vi "PayneHW1.vi"() -> ()   [LabVIEW 2011]
panel:
  out "Units":string
  in  "stop":bool
  in  "Unit Selector":u16(ring) items=["Celsius", "Kelvin", "Fahrenheit"]
  in  "Voltage":dbl(slide) scale=0.0..4.0
  out "Temperature":dbl(slide) scale=-350.0..600.0
  out "Invalid Range Danger":bool
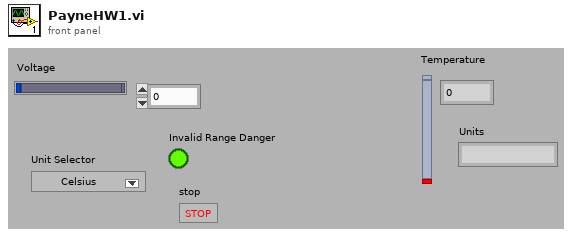
[diagram p1: front panel]
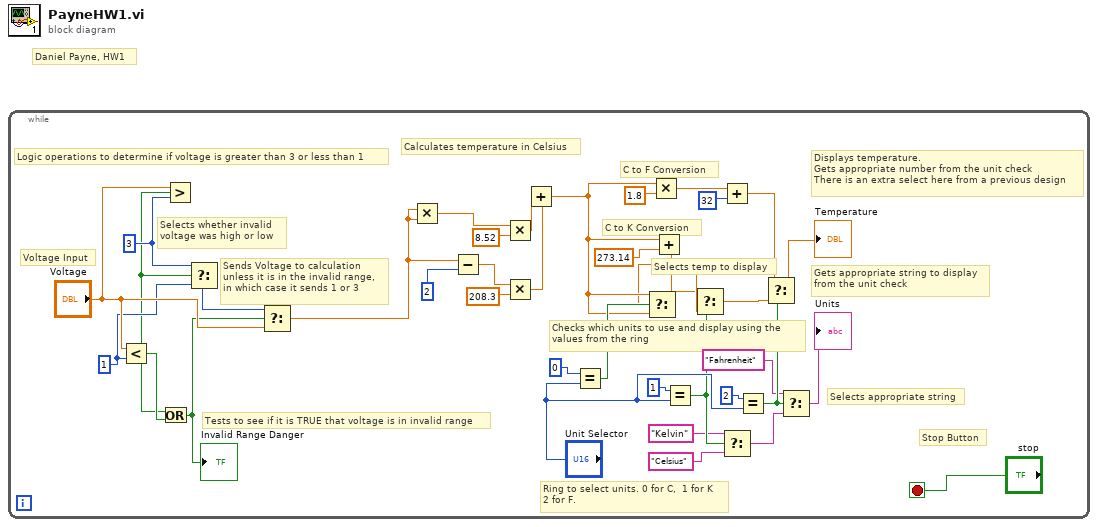
[diagram p0: block diagram]
diagram:
  # "Daniel Payne, HW1"
  n1 = while {
    stop <- "stop" stop-if-true
    w26 = 3
    w25 = 1
    # "Selects temp to display"
    # "C to F Conversion"
    # "C to K Conversion"
    # "Stop Button"
    # "Selects appropriate string"
    # "Displays temperature. \nGets appropriate number from the unit check \nThere is an extra select here from a previous design"
    # "Gets appropriate string to display\nfrom the unit check"
    # "Checks which units to use and display using the\nvalues from the ring"
    # "Ring to select units. 0 for C,  1 for K\n2 for F."
    # "Calculates temperature in Celsius"
    # "Selects whether invalid \nvoltage was high or low"
    # "Sends Voltage to calculation\nunless it is in the invalid range, \nin which case it sends 1 or 3"
    # "Tests to see if it is TRUE that voltage is in invalid range"
    # "Logic operations to determine if voltage is greater than 3 or less than 1"
    # "Voltage Input"
    n2 = Less?(x="Voltage", y=w25) -> (x < y?=w38:bool)
    n3 = Greater?(x="Voltage", y=w26) -> (0:w24:bool)
    n4 = Or(x=w24, y=w38) -> (x .or. y?=w29:bool)
    "Invalid Range Danger" <- w29
    n5 = Select(t=w26, s=w24, f=w25) -> (s? t:f=w27:i32)
    n6 = Select(t=w27, s=w29, f="Voltage") -> (s? t:f=w28:dbl)
    n7 = Multiply(x=w28, y=w28) -> (x*y=w34:dbl)
    n8 = Subtract(x=w28, y=2) -> (x-y=w36:dbl)
    n9 = Multiply(x=w34, y=8.52) -> (x*y=w31:dbl)
    n10 = Multiply(x=w36, y=208.3) -> (x*y=w32:dbl)
    n11 = Add(x=w31, y=w32) -> (x+y=w14:dbl)
    n12 = Equal?(x=0, y="Unit Selector") -> (x = y?=w20:bool)
    n13 = Select(t=w14, s=w20, f=w14) -> (s? t:f=w13:dbl)
    n14 = Multiply(x=w14, y=1.8) -> (x*y=w16:dbl)
    n15 = Add(x=w14, y=273.14) -> (x+y=w12:dbl)
    n16 = Equal?(x=1, y="Unit Selector") -> (x = y?=w8:bool)
    n17 = Select(t=w12, s=w8, f=w13) -> (s? t:f=w11:dbl)
    n18 = Add(x=w16, y=32) -> (x+y=w10:dbl)
    n19 = Select(t="Kelvin", s=w8, f="Celsius") -> (s? t:f=w5:string)
    n20 = Equal?(x=2, y="Unit Selector") -> (x = y?=w4:bool)
    n21 = Select(t=w10, s=w4, f=w11) -> (s? t:f=→"Temperature":dbl)
    n22 = Select(t="Fahrenheit", s=w4, f=w5) -> (s? t:f=→"Units":string)
  }
